vi "example_usb.vi"() -> ()   [LabVIEW 2025, in "libirimager_direct_binding.lvlib"]
uses:
  GitHub/In-situ-monitoring-of-powder-bed-fusion-additive-manufacturing/system_development/Orichalcum/v0.2/Software_design/thermal-camera/VI/libirimager_direct_binding.lvlib
panel:
  in  "stop":bool
  in  "Focus Pos %":sgl min=0 max=100
  in  "setFocusPos":bool
  out "function return setFocusPos":i32
  out "function return set radiation":i32
  in  "tAmbient":sgl=-999.9 format="%#_6f"
  in  "transmissivity(0..1)":sgl=1.0 format="%#_6f"
  in  "emissivity(0..1)":sgl=1.0 format="%#_6f"
  in  "setRadiation":bool
  in  "STOP":bool
  out "Thermal Image":picture
  out "function return thm":i32
  out "thermal data out":u16[](array[numeric])
  out "function return savepng":i32
  in  "triggerFlag":bool
  out "function return triggerAutoflag":i32
  in  "set_trigger_mode":bool
  in  "state":i32
  out "function return setAutoflag":i32
  in  "terminate":bool
  out "function return terminate":i32
  in  "getThm":bool
  in  "connect_usb":bool
  in  "xml_camera_config":string="generic.xml"
  out "function return":i32
  out "w out":i32
  out "h out":i32
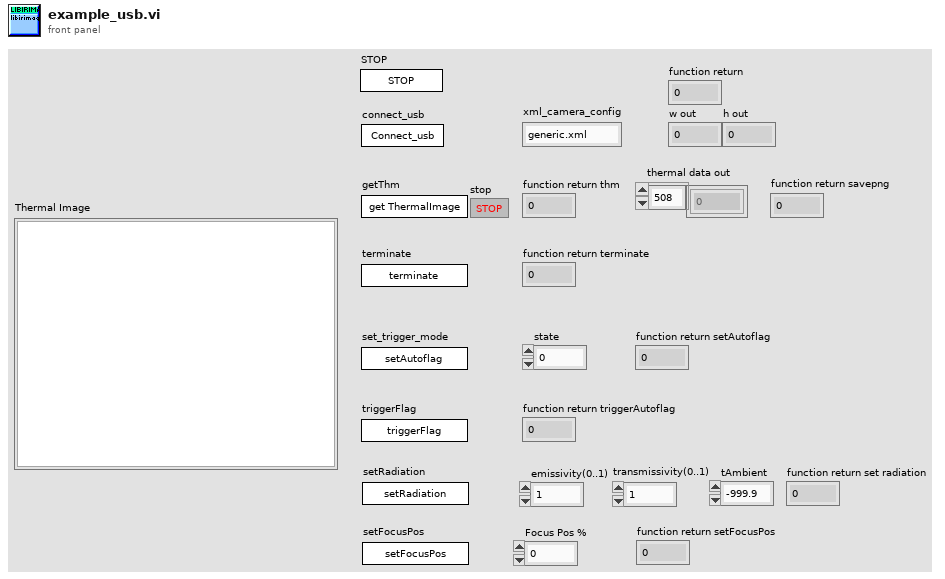
[diagram p1: front panel]
types:
  T1 = typedef "imagedata.ctl" = cluster{"image type":i32, "image depth":i32, "image":u8[], "mask":u8[], "colors":u32[], "Rectangle":cluster{"left":i16, "top":i16, "right":i16, "bottom":i16}}
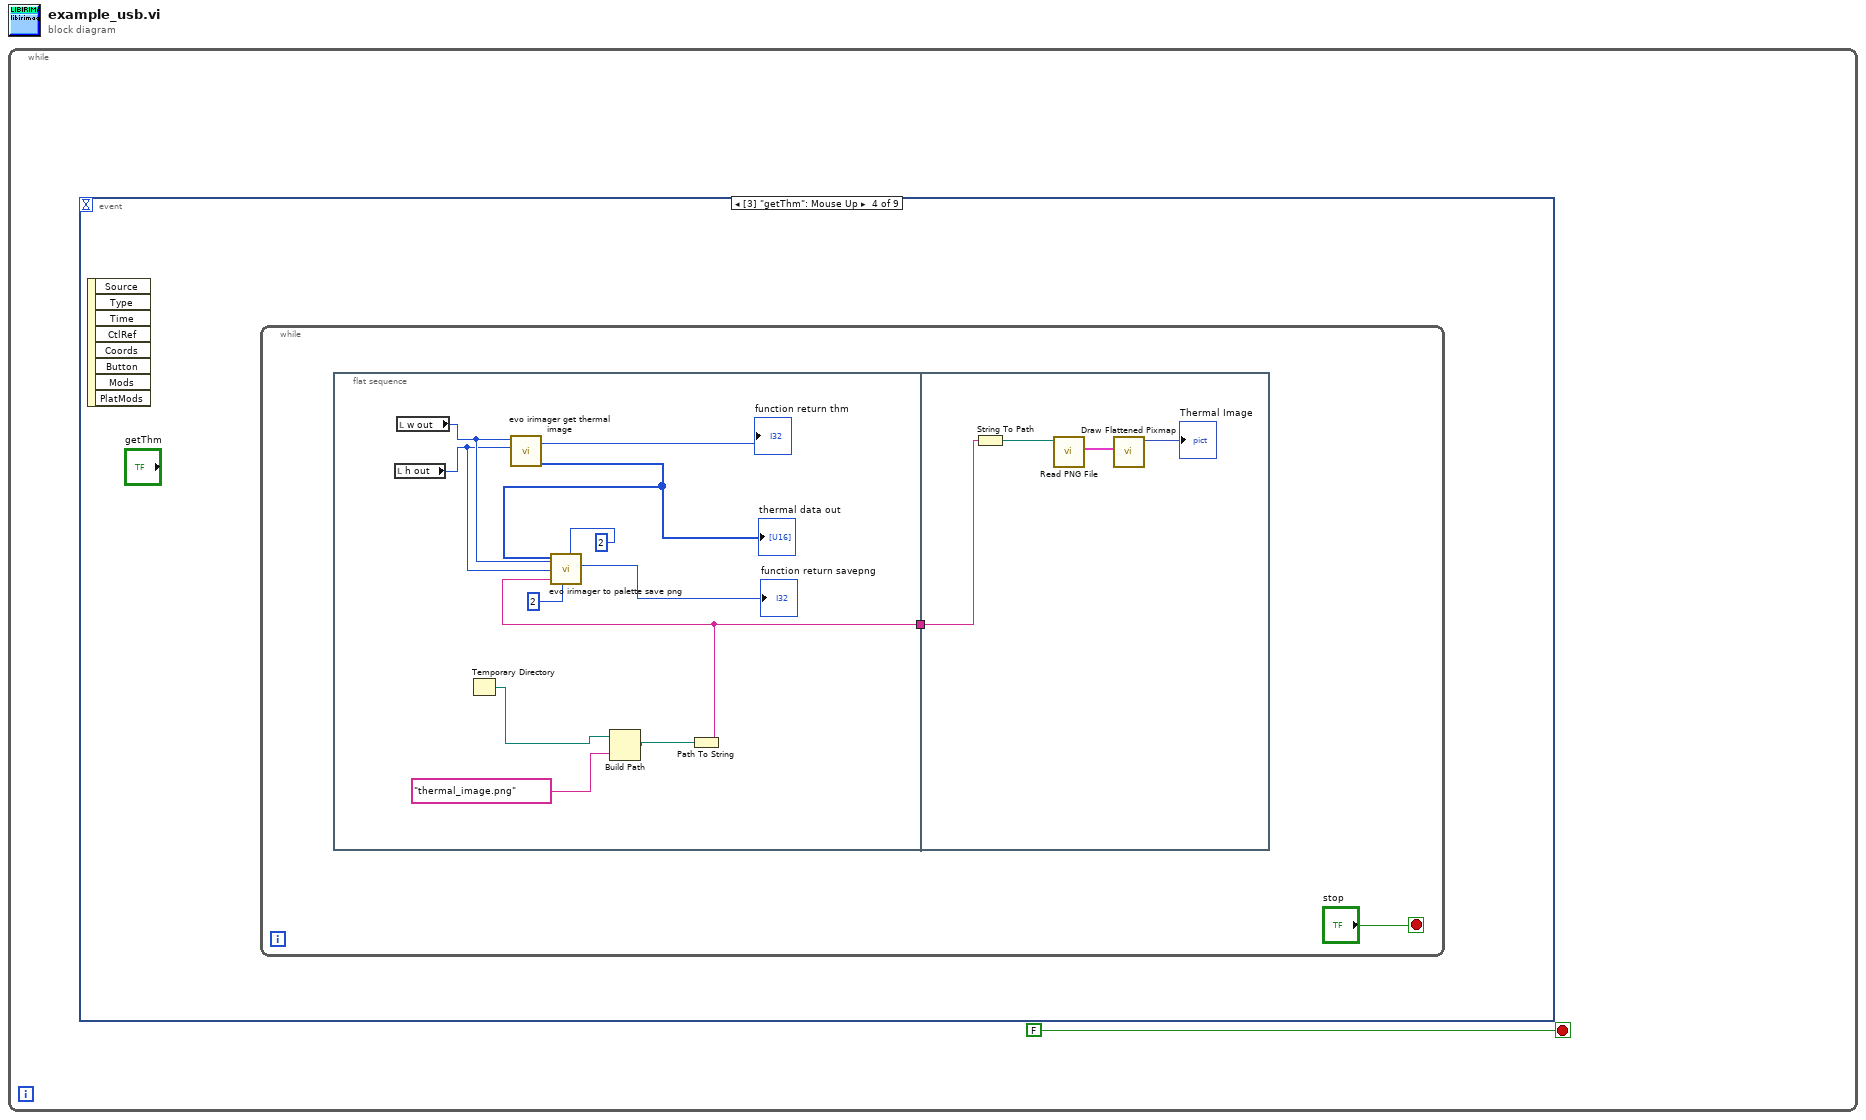
[diagram p0: block diagram]
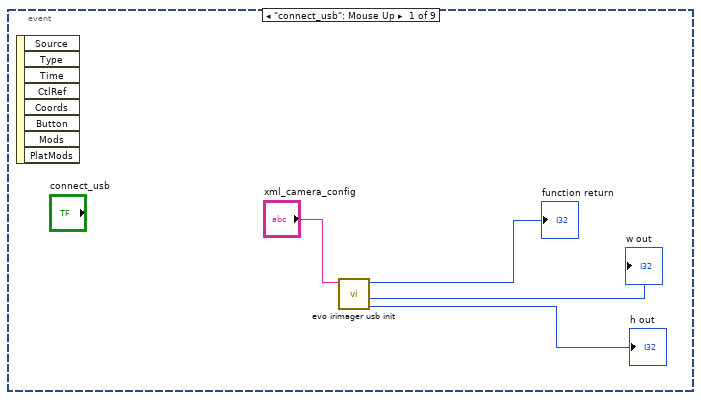
[diagram p2: hidden frame]
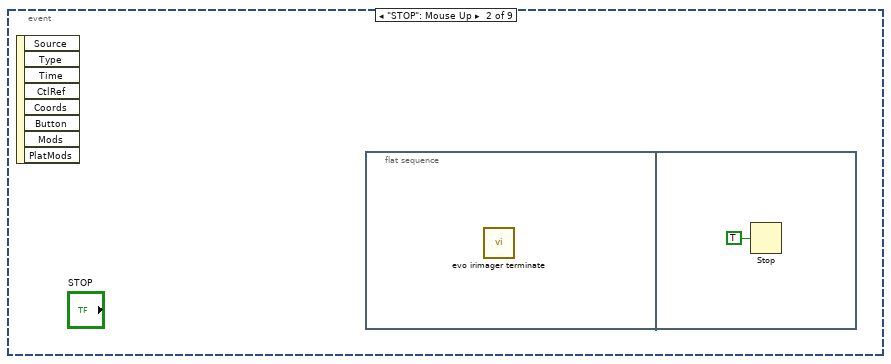
[diagram p3: hidden frame]
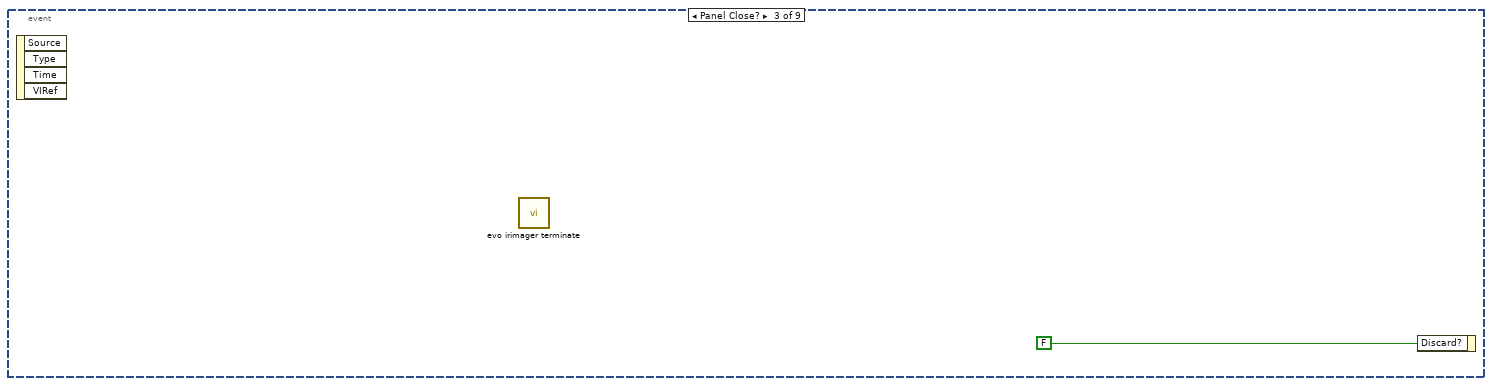
[diagram p4: hidden frame]
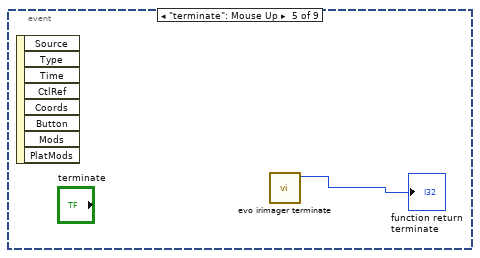
[diagram p5: hidden frame]
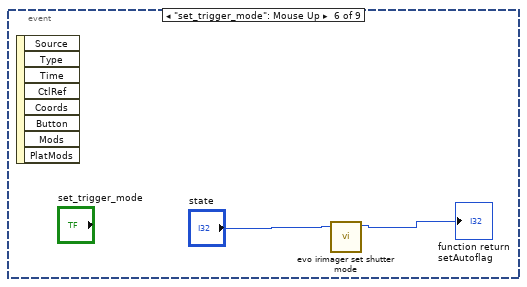
[diagram p6: hidden frame]
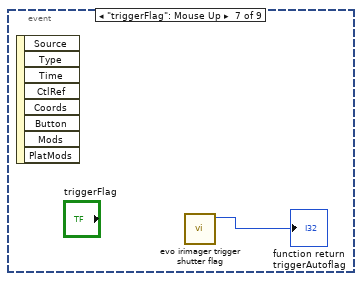
[diagram p7: hidden frame]
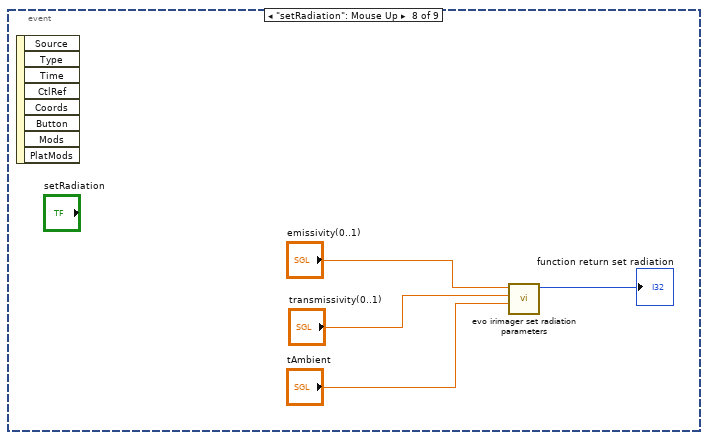
[diagram p8: hidden frame]
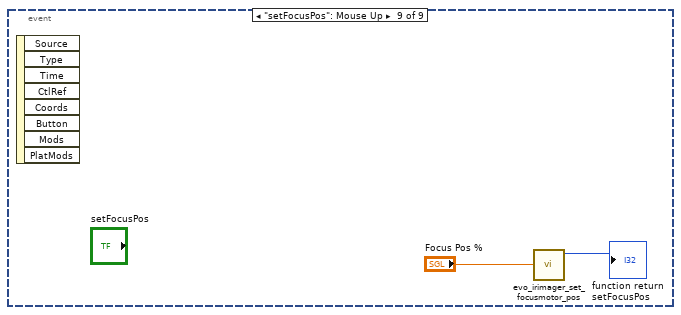
[diagram p9: hidden frame]
diagram:
  n1 = while {
    stop <- FALSE stop-if-true
    n2 = event shown="[3] \"getThm\": Mouse Up" {
      selector: _ -> [_ _ _ _ _ _ _ _ _]
      dyn-events: _ -> [_ _ _ _ _ _ _ _ _]
      timeout: _ -> [_ _ _ _ _ _ _ _ _]
      event "connect_usb": Mouse Up {
        n3 = event-data() -> ()  [unwired: 1 in, 8 out]
        n4 = call "evo irimager usb init.vi"("xml_config"="xml_camera_config") -> ("h out"=→"h out":i32, "w out"=→"w out":i32, "function return 2"=→"function return":i32)  [unwired: 7 in, 1 out]
      }
      event "STOP": Mouse Up {
        n5 = event-data() -> ()  [unwired: 1 in, 8 out]
        n6 = flat-sequence {
          frame #0 {
            n7 = call "evo irimager terminate.vi"() -> ()  [unwired: 11 in, 1 out]
          }
          frame #1 {
            n8 = Stop(stop? (T)=TRUE ("Stopp? (T)")) -> ()
          }
        }
      }
      event Panel Close? {
        n9 = event-data() -> ()  [unwired: 1 in, 4 out]
        n10 = call "evo irimager terminate.vi"() -> ()  [unwired: 11 in, 1 out]
        n11 = event-data("Discard?"=FALSE ("Verwerfen?")) -> ()  [unwired: 1 in, 1 out]
      }
      event "getThm": Mouse Up {
        n12 = event-data() -> ()  [unwired: 1 in, 8 out]
        n13 = while {
          stop <- "stop" stop-if-true
          n14 = flat-sequence {
            tunnel: [w12] -> w9
            tunnel: w9 -> [w21]
            frame #0 {
              n15 = local read "h out"() -> (w17:i32)
              n16 = local read "w out"() -> (w18:i32)
              n17 = Temporary Directory() -> (w11:path)
              n18 = call "evo irimager get thermal image.vi"("h"=w17, "w"=w18) -> ("data out"=w19:u16[], "function return"=→"function return thm":i32)  [unwired: 6 in, 2 out]
              "thermal data out" <- w19
              n19 = Build Path(base path=w11, name or relative path="thermal_image.png" ("String")) -> (appended path=w10:path)
              n20 = Path To String(path=w10) -> (string=w12:string)
              n21 = call "evo irimager to palette save png.vi"("palette_scale"=2, "palette"=2, "path"=w12, "h"=w17, "w"=w18, "thermal_data"=w19) -> ("function return"=→"function return savepng":i32)  [unwired: 4 in, 1 out]
            }
            frame #1 {
              n22 = String To Path(string=w21) -> (path=w22:path)
              n23 = call <vilib>:"Read PNG File.vi"("path to PNG file"=w22) -> ("image data"=w23:T1)  [unwired: 8 in, 2 out]
              n24 = call <vilib>:"Draw Flattened Pixmap.vi"("image data"=w23) -> ("new picture"=→"Thermal Image":picture)  [unwired: 8 in]
            }
          }
        }
      }
      event "terminate": Mouse Up {
        n25 = event-data() -> ()  [unwired: 1 in, 8 out]
        n26 = call "evo irimager terminate.vi"() -> ("function return"=→"function return terminate":i32)  [unwired: 11 in]
      }
      event "set_trigger_mode": Mouse Up {
        n27 = event-data() -> ()  [unwired: 1 in, 8 out]
        n28 = call "evo irimager set shutter mode.vi"("mode"="state") -> ("function return"=→"function return setAutoflag":i32)  [unwired: 10 in]
      }
      event "triggerFlag": Mouse Up {
        n29 = event-data() -> ()  [unwired: 1 in, 8 out]
        n30 = call "evo irimager trigger shutter flag.vi"() -> ("function return"=→"function return triggerAutoflag":i32)  [unwired: 11 in]
      }
      event "setRadiation": Mouse Up {
        n31 = event-data() -> ()  [unwired: 1 in, 8 out]
        n32 = call "evo irimager set radiation parameters.vi"("tAmbient"="tAmbient", "transmissivity"="transmissivity(0..1)", "emissivity"="emissivity(0..1)") -> ("function return"=→"function return set radiation":i32)  [unwired: 8 in]
      }
      event "setFocusPos": Mouse Up {
        n33 = event-data() -> ()  [unwired: 1 in, 8 out]
        n34 = call "evo_irimager_set_focusmotor_pos.vi"("Focus Pos %"="Focus Pos %") -> ("function return"=→"function return setFocusPos":i32)  [unwired: 10 in]
      }
    }
  }
